vi "1. JKISM vs CSM.vi"() -> ()   [LabVIEW 2017]
doc: "### 1. JKISM vs CSM.vi\n\n#### Overview\n\nCSM 是仿照 JKISM 逻辑设计的 LabVIEW 程序开发框架，两个框架都使用基于字符串的消息队列来实现核心逻辑。本示例用于演示CSM基于JKISM的拓展。\n\n#### Introduction\n\n本示例比较 JKISM 框架和 CSM 框架之间的代码。两个框架都使用基于字符串的消息队列来实现核心状态机。\n\n#### Steps\n\n基于 JKISM，CSM 具有以下主要扩展功能，让我们逐步解释：\n\n- Step1: CSM是一个程序框架因此它需要模块的名称\n- Step2：重新设计了核心字符串解析引擎。\n- Step2.1 JKISM 使用 Parse State Queue.vi，它只输出下一个状态队列及其对应的参数（位于 >> 之后），主要用作“出队元素”。\n- Step2.2 CSM 使用 Parse State Queue++.vi 额外添加了以下主要功能：\n \\- 基于状态队列输入自动创建/处理/销毁队列/用户事件机制，因此用户只需给出相应的高级字符串消息。\n \\- 模块间/VI 间的消息可以被传输。\n \\- 额外的输入，如 Dequeue Timeout、Response Timeout 和 Allowed Messages，用于实现更高级的功能。\n- Step3：CSM 添加了一个内部状态调试日志 history.vi 用于更好的调试和记录，状态历史可以直接显示在前面板上。\n- Step4：CSM 定义了一系列字符串语法来实现本地/模块间消息传输，例如同步消息、异步消息、状态创建/注册/注销等。\n- Step4.1: JKISM 只定义了本地状态的轮转。它可以携带一个参数以及注释。\n- Step4.2: CSM是一个软件框架，因此它定义了模块。以及模块之间的消息通讯。\n- Step5: CSM 定义了一些基础的状态，用于处理模块之间通讯的逻辑行为。\n- Step5.1: \"Critical Error\" 用于处理一些无法恢复的错误。\n- Step5.2: \"Target Timeout Error\" 用于处理模块消息通讯超时的错误。\n- Step5.3: \"Target Error\" 用于处理模块不存在的错误。\n- STEP5.4: \"Async Response\" 用于处理异步消息的回复。\n- Step5.5：”Response\" 用于处理同步消息的回复。\n- Step5.6: \"Async Message Posted\" 用于处理异步消息发送后的操作。\n- Step5.7:(optional) \"Events: Register\" 和 \"Events: Unregister\" 中使用的消息事件，用于触发带有Event Structure的CSM模块跳出。\n- Step5.7:(optional) \"<New State Notifier Event>\" 配合Step5.7实现在外部消息到来后，跳出事件结构等待\n- Step5.8:(optional) CSM推荐使用 API 分组提供对外的接口，但是实际上所有的分支都可以使用消息调用。\n- Step6. CSM额外定义了\"Msg/Rsp's CSM\" 用于定位外部消息、状态的来源模块\n- Step7. 额外的消息信息，如Response的源消息名称、源参数等，可以由此获得。\n- Step8. CSM 预置了消息返回.\n- Step9：CSM 扩展了调试工具，详情请参阅选板 CSM->CSM Debug Tools。"
uses:
  user.lib/_NEVSTOP/Communicable State Machine(CSM)/AdvanceAPI/CSM - Revert Arguments-Safe String.vi
  user.lib/_NEVSTOP/Communicable State Machine(CSM)/AdvanceAPI/CSM - Make String Arguments Safe.vi
  user.lib/_NEVSTOP/Communicable State Machine(CSM)/AdvanceAPI/CSM - Break Down Multiple States String.vi
  user.lib/_NEVSTOP/Communicable State Machine(CSM)/AdvanceAPI/CSM - Compact Multiple States.vi
  user.lib/_NEVSTOP/Communicable State Machine(CSM)/AdvanceAPI/CSM - Keywords.vi
  user.lib/_NEVSTOP/Communicable State Machine(CSM)/_Shared/Trim Single-line Text.vi
  user.lib/_NEVSTOP/Communicable State Machine(CSM)/Communicable State Machine.lvlib
panel:
  out "State History":string
  in  "Exit":bool
  # "#CSM-Example Overview\n\nCSM 是仿照 JKISM 逻辑设计的 LabVIEW 程序开发框架，两个框架都使用基于字符串的消息队列来实现核心逻辑。本示例用于演示CSM基于JKISM的拓展。"
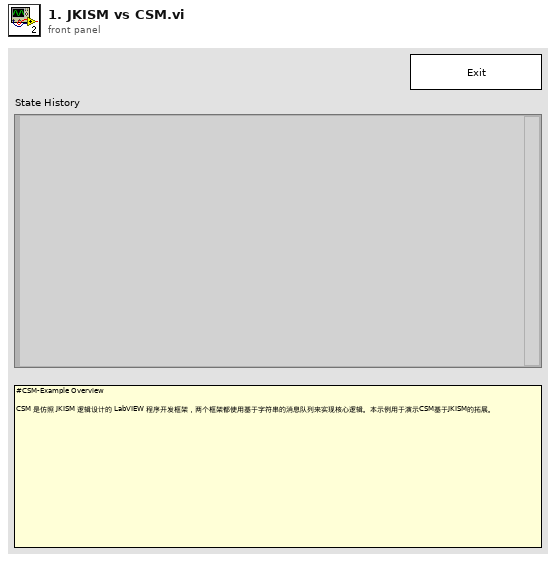
[diagram p1: front panel]
types:
  T1 = enum32{"Invalid", "Standard", "Closed", "Hidden", "Minimized", "Maximized"}
  T2 = enum32{"invalid app kind", "Development System", "Run Time System", "Student Edition", "Embedded LabVIEW", "Evaluation", "Custom"}
  T3 = cluster{"Core":cluster{"Current VI Reference":refnum<vi>, "Close Panel on Exit?":bool}, "Your Boolean data":bool, "Your string data":string}
  T4 = cluster{"Current VI Reference":refnum<vi>, "Close Panel on Exit?":bool}
  T5 = typedef "Communicable State Machine.lvlib/_CSM_Response Source Message.ctl" = cluster{"‘State":string, "’Arguments":string, "’Error":errorcluster}
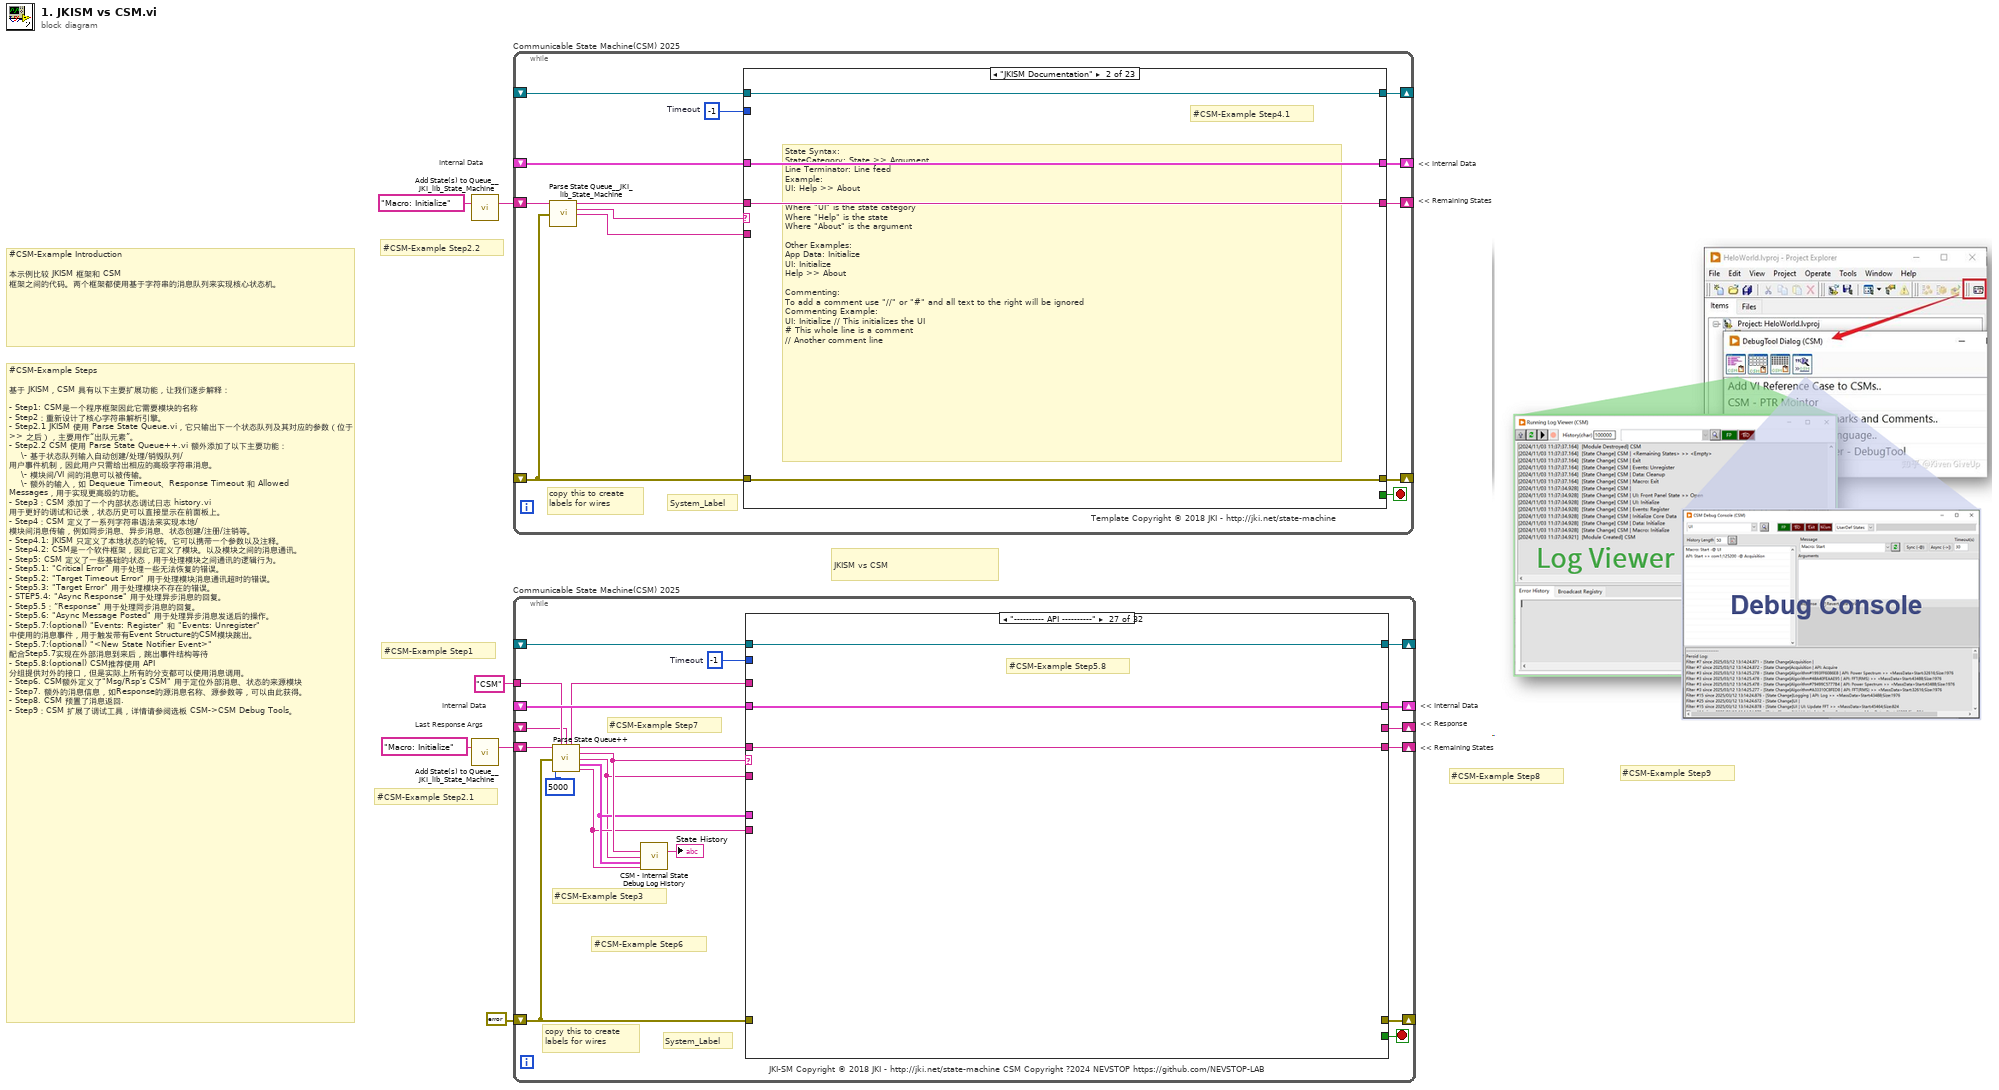
[diagram p0: block diagram]
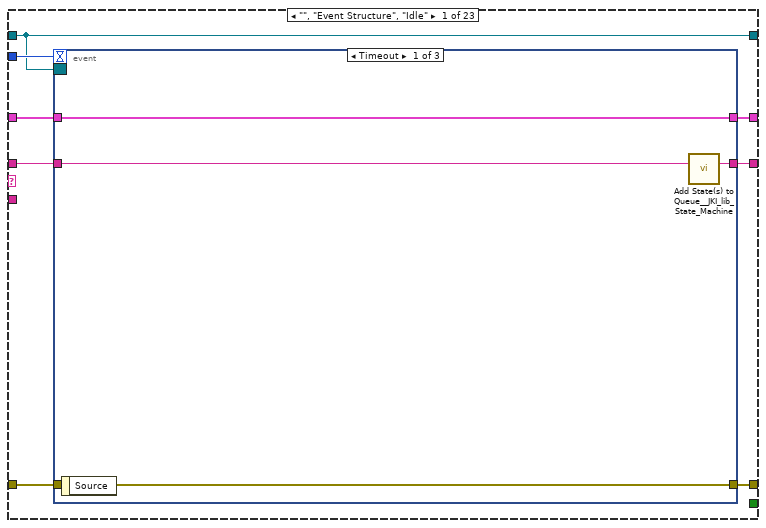
[diagram p2: hidden frame]
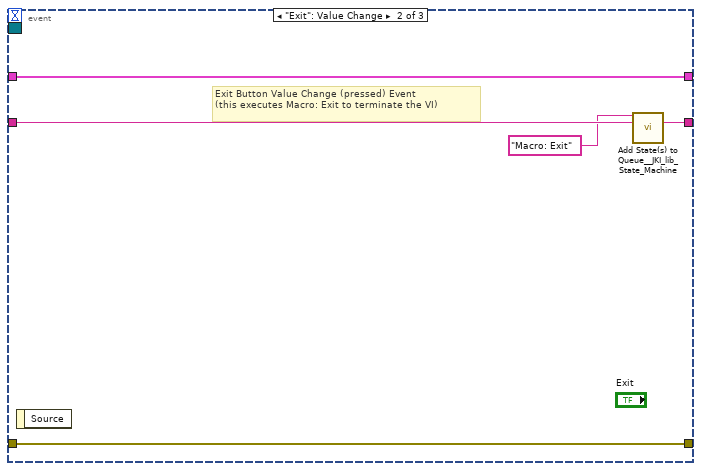
[diagram p3: hidden frame]
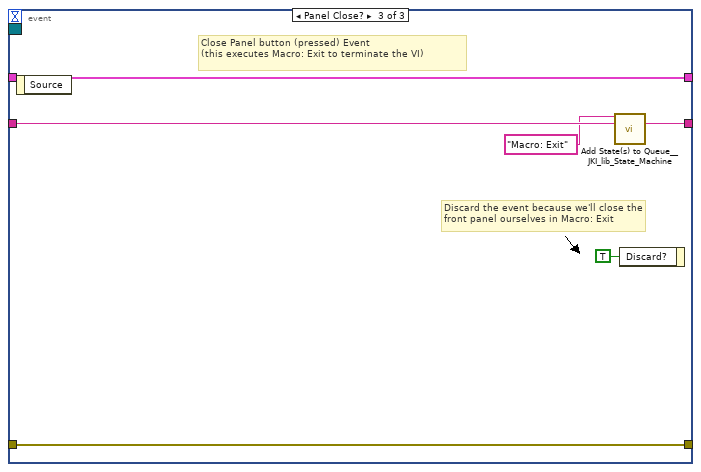
[diagram p4: hidden frame]
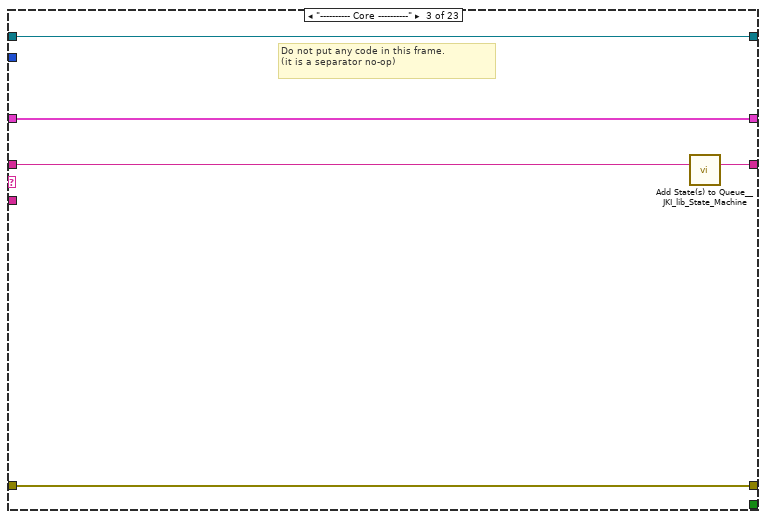
[diagram p5: hidden frame]
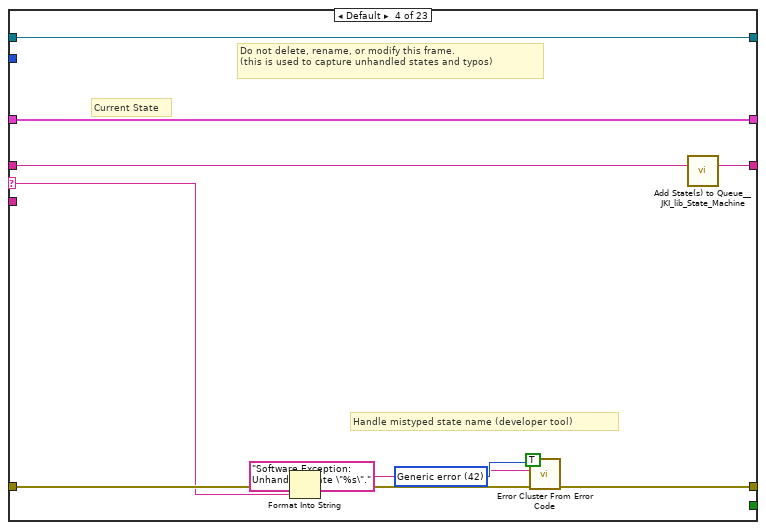
[diagram p6: hidden frame]
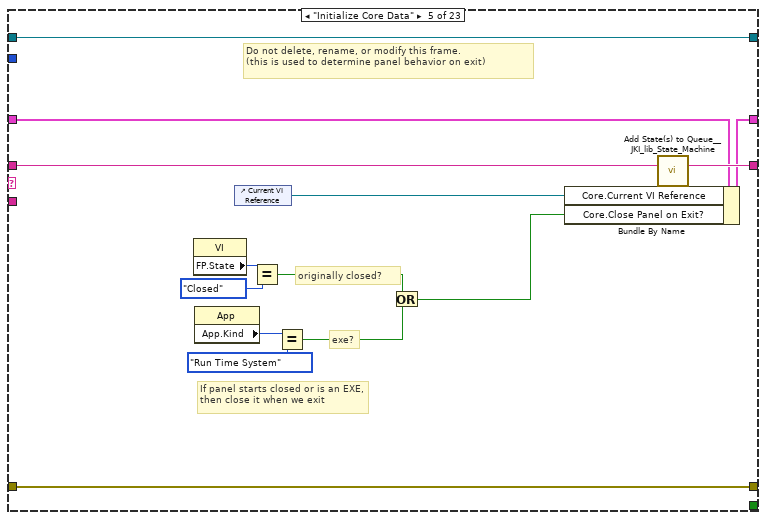
[diagram p7: hidden frame]
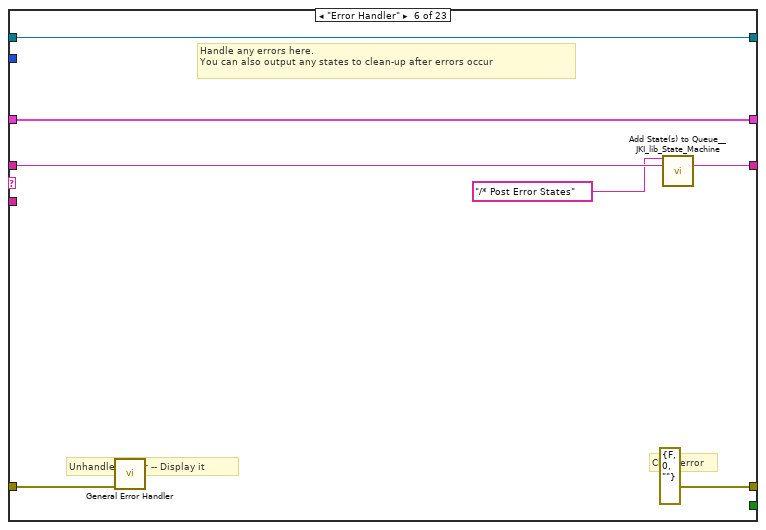
[diagram p8: hidden frame]
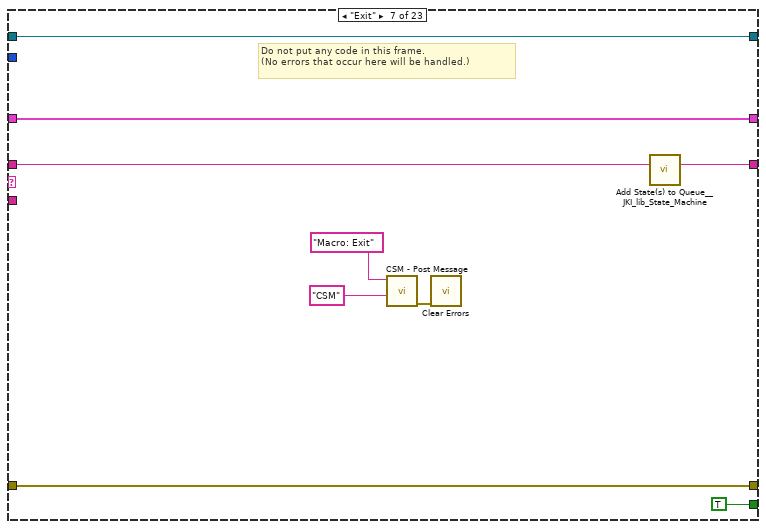
[diagram p9: hidden frame]
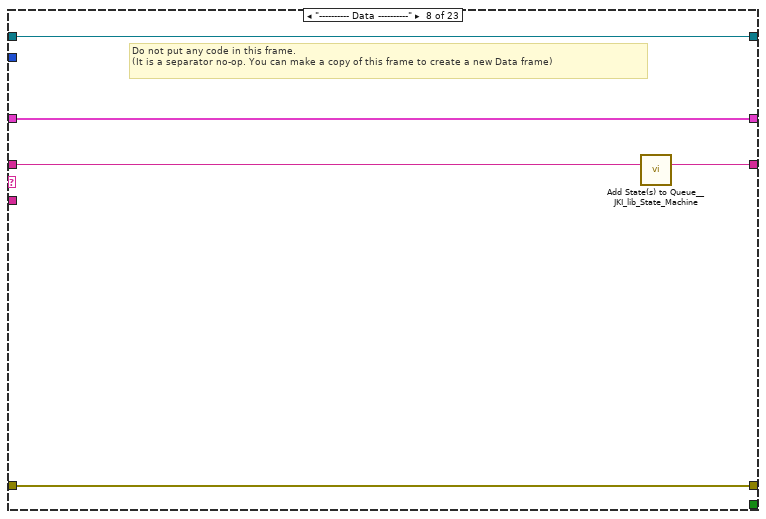
[diagram p10: hidden frame]
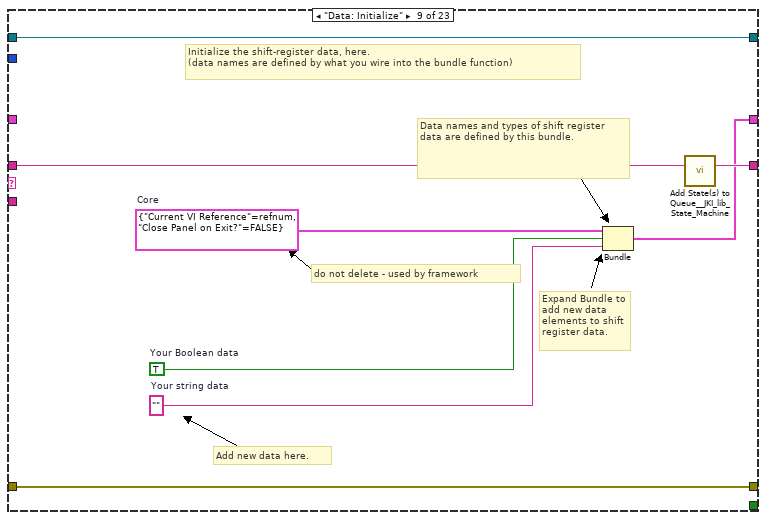
[diagram p11: hidden frame]
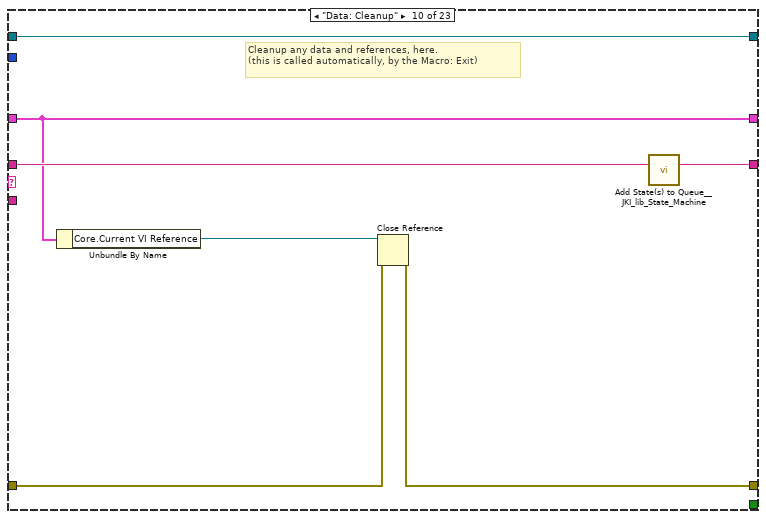
[diagram p12: hidden frame]
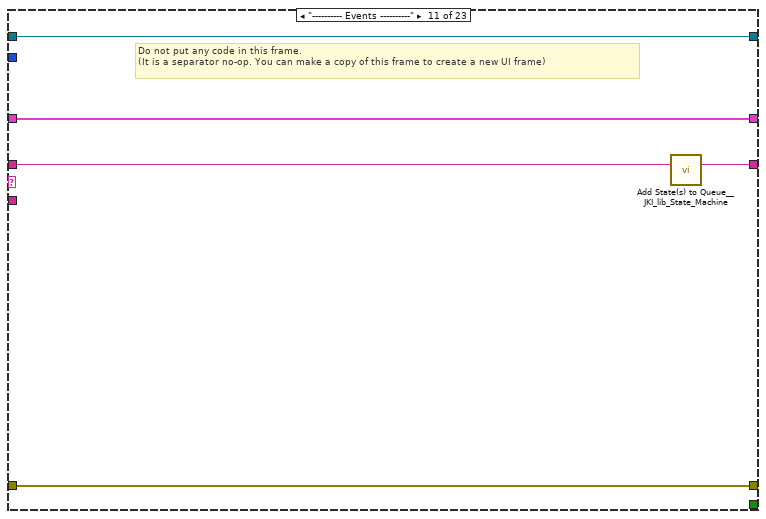
[diagram p13: hidden frame]
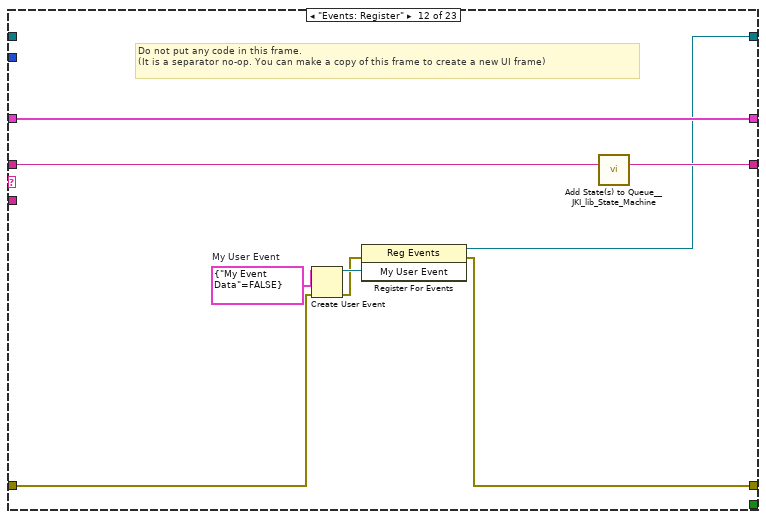
[diagram p14: hidden frame]
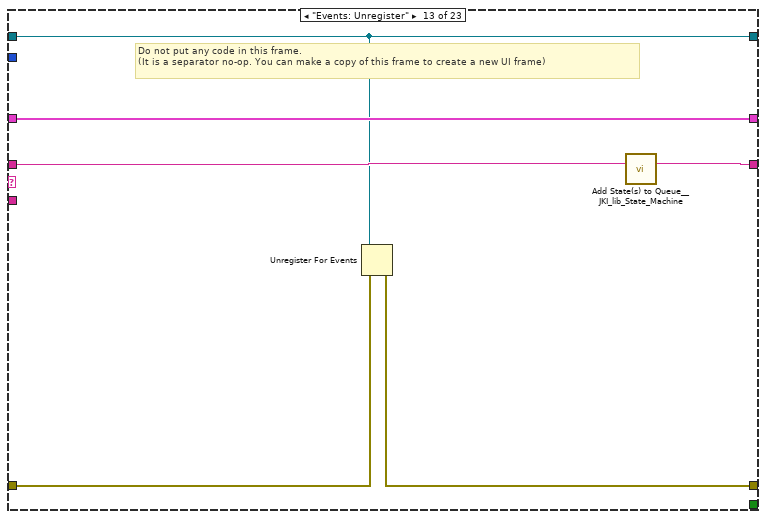
[diagram p15: hidden frame]
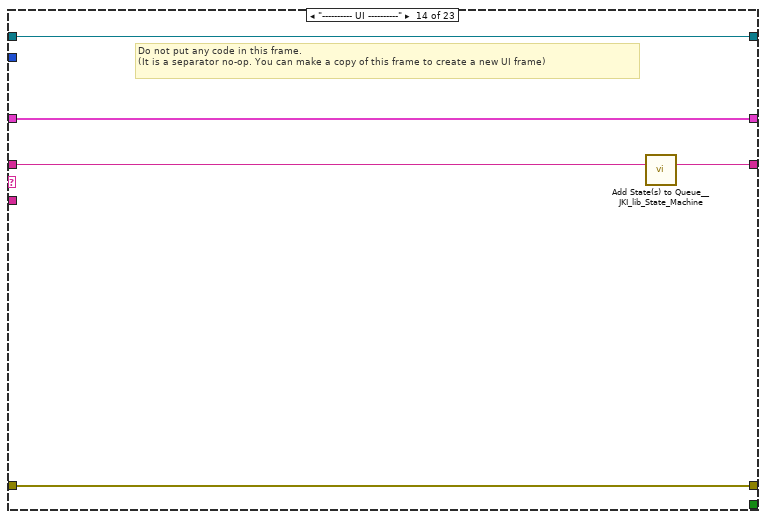
[diagram p16: hidden frame]
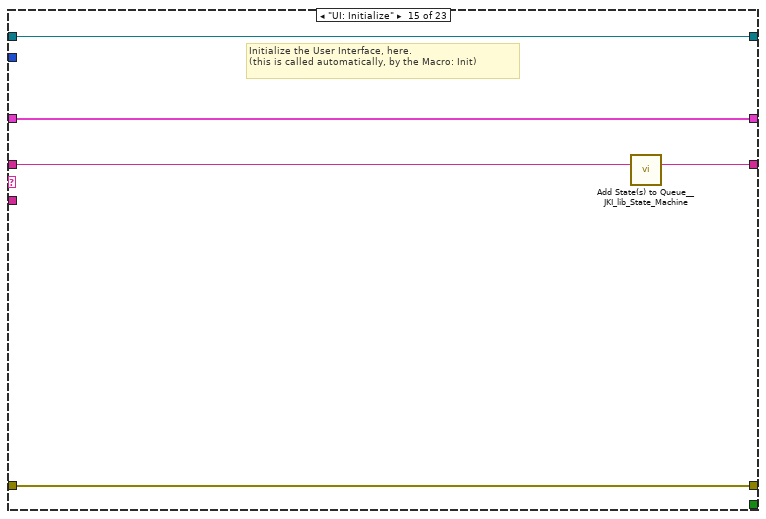
[diagram p17: hidden frame]
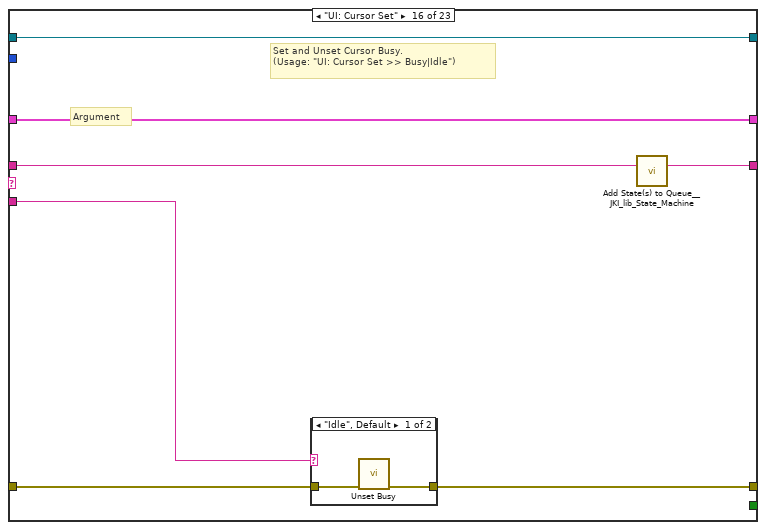
[diagram p18: hidden frame]
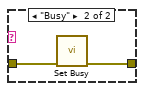
[diagram p19: hidden frame]
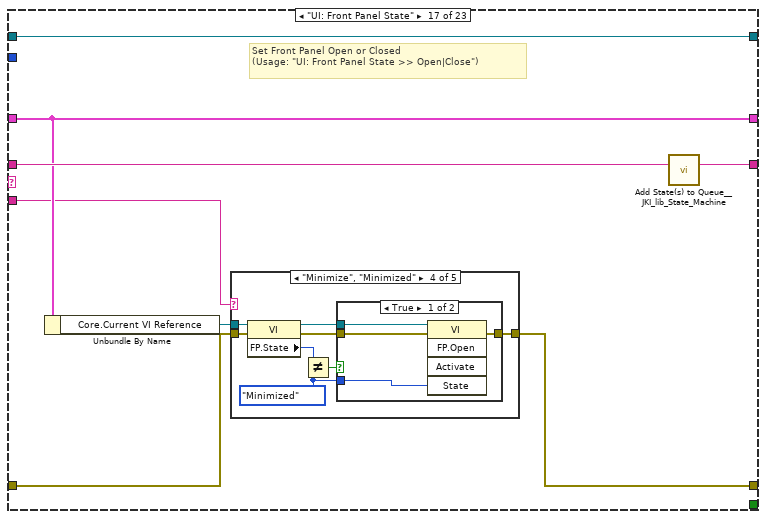
[diagram p20: hidden frame]
diagram:
  # "#CSM-Example Step9"
  # "#CSM-Example Step8"
  # "#CSM-Example Step2.2"
  # "#CSM-Example Step2.1"
  # "#CSM-Example Step1"
  # "#CSM-Example Steps\n\n基于 JKISM，CSM 具有以下主要扩展功能，让我们逐步解释：\n\n- Step1: CSM是一个程序框架因此它需要模块的名称\n- Step2：重新设计了核心字符串解析引擎。\n- Step2.1 JKISM 使用 Parse State Queue.vi，它只输出下一个状态队列及其对应的参数（位于 >> 之后），主要用作“出队元素”。\n- Step2.2 CSM 使用 Parse State Queue++.vi 额外添加了以下主要功能：\n    \\- 基于状态队列输入自动创建/处理/销毁队列/用户事件机制，因此用户只需给出相应的高级字符串消息。\n    \\- 模块间/VI 间的消息可以被传输。\n    \\- 额外的输入，如 Dequeue Timeout、Response Timeout 和 Allowed Messages，用于实现更高级的功能。\n- Step3：CSM 添加了一个内部状态调试日志 history.vi 用于更好的调试和记录，状态历史可以直接显示在前面板上。\n- Step4：CSM 定义了一系列字符串语法来实现本地/模块间消息传输，例如同步消息、异步消息、状态创建/注册/注销等。\n- Step4.1: JKISM 只定义了本地状态的轮转。它可以携带一个参数以及注释。\n- Step4.2: CSM是一个软件框架，因此它定义了模块。以及模块之间的消息通讯。\n- Step5: CSM 定义了一些基础的状态，用于处理模块之间通讯的逻辑行为。\n- Step5.1: \"Critical Error\" 用于处理一些无法恢复的错误。\n- Step5.2: \"Target Timeout Error\" 用于处理模块消息通讯超时的错误。\n- Step5.3: \"Target Error\" 用于处理模块不存在的错误。\n- STEP5.4: \"Async Response\" 用于处理异步消息的回复。\n- Step5.5：”Response\" 用于处理同步消息的回复。\n- Step5.6: \"Async Message Posted\" 用于处理异步消息发送后的操作。\n- Step5.7:(optional) \"Events: Register\" 和 \"Events: Unregister\" 中使用的消息事件，用于触发带有Event Structure的CSM模块跳出。\n- Step5.7:(optional) \"<New State Notifier Event>\" 配合Step5.7实现在外部消息到来后，跳出事件结构等待\n- Step5.8:(optional) CSM推荐使用 API 分组提供对外的接口，但是实际上所有的分支都可以使用消息调用。\n- Step6. CSM额外定义了\"Msg/Rsp's CSM\" 用于定位外部消息、状态的来源模块\n- Step7. 额外的消息信息，如Response的源消息名称、源参数等，可以由此获得。\n- Step8. CSM 预置了消息返回.\n- Step9：CSM 扩展了调试工具，详情请参阅选板 CSM->CSM Debug Tools。"
  # "#CSM-Example Introduction\n\n本示例比较 JKISM 框架和 CSM 框架之间的代码。两个框架都使用基于字符串的消息队列来实现核心状态机。"
  # "JKISM vs CSM"
  # "<< Internal Data"
  # "<< Remaining States"
  # "Internal Data"
  # "Last Response Args"
  # "Internal Data"
  # "<< Internal Data"
  # "<< Response"
  # "<< Remaining States"
  n1 = call <vilib>:"Add State(s) to Queue__JKI_lib_State_Machine.vi"("State(s) in (\"\")"="Macro: Initialize") -> ("States Out"=w6:string)  [unwired: 14 in]
  n2 = call <vilib>:"Add State(s) to Queue__JKI_lib_State_Machine.vi"("State(s) in (\"\")"="Macro: Initialize" ("Init State(\"Macro: Initialize\")")) -> ("States Out"=w1:string)  [unwired: 14 in]
  n3 = while "Communicable State Machine(CSM) 2025" {
    shift-right: [w12] -> _
    shift-left: _ -> [w11]
    shift-right: [w15] -> _
    shift-left: _ -> [w9]
    shift-right: [w14] -> _
    shift-left: w6 -> [w16]
    shift-right: [w8] -> _
    shift-left: _ -> [w7]
    stop <- w13 stop-if-true
    w10 = -1  # Timeout
    # "copy this to create labels for wires"
    # "System_Label"
    # "Template Copyright © 2018 JKI - http://jki.net/state-machine"
    n4 = call <vilib>:"Parse State Queue__JKI_lib_State_Machine.vi"("State Queue"=w16, "Error In (no error)"=w9) -> ("Remaining States"=w18:string, "Current State"=w19:string, "Arguments"=w17:string)  [unwired: 11 in]
    n5 = case shown="\"JKISM Documentation\"" w19 {
      selector: w19 -> [_ _ _ w53 _ _ _ _ _ _ _ _ _ _ _ _ _ _ _ _ _ _ _]
      tunnel: w18 -> [w27 w44 w51 w57 w77 w84 w93 w98 w106 w113 w118 w127 w133 w138 w143 w150 w162 w232 w238 w249 w254 w259 w264]
      tunnel: w17 -> [_ _ _ _ _ _ _ _ _ _ _ _ _ _ _ w145 w156 _ _ _ _ _ _]
      tunnel: w11 -> [w25 w45 w48 w55 w70 w81 w91 w95 _ w108 w115 w125 w131 w135 w141 w148 w158 w229 w235 w246 w251 w256 w261]
      tunnel: [w24 w43 w49 w59 w74 errorcluster {"status"=FALSE, "code"=0, "source"=""} ("error out") w90 w96 w103 w109 w116 w119 w128 w136 w140 w146 w159 w230 w236 w247 w252 w257 w262] -> w15
      tunnel: w9 -> [w23 w43 w49 w58 w74 w80 w90 w96 w103 w110 w116 w121 w129 w136 w140 w147 w160 w230 w236 w247 w252 w257 w262]
      tunnel: [w26 w44 w50 w56 w76 w83 w92 w97 w105 w112 w117 w126 w132 w137 w142 w149 w161 w231 w237 w248 w253 w258 w263] -> w14
      tunnel: [_ _ _ _ _ _ TRUE _ _ _ _ _ _ _ _ _ _ _ _ _ _ _ _] -> w13
      tunnel: [w22 w45 w48 w55 w75 w81 w91 w95 w104 w108 w115 w125 w131 w135 w141 w148 w158 w229 w235 w246 w251 w256 w261] -> w12
      tunnel: w10 -> [w21 _ _ _ _ _ _ _ _ _ _ _ _ _ _ _ _ _ _ _ _ _ _]
      tunnel: [w20 w46 w47 w52 w64 w78 w88 w94 w99 w107 w114 w122 w130 w134 w139 w144 w155 w228 w233 w239 w250 w255 w260] -> w8
      tunnel: w7 -> [w20 w46 w47 w52 w64 w78 w88 w94 w99 w107 w114 _ w130 w134 w139 w144 w155 w228 w233 w239 w250 w255 w260]
      frame "", "Event Structure", "Idle" {
        n6 = event shown="[0] Timeout" {
          selector: w20 -> [_ _ _]
          dyn-events: _ -> [_ _ _]
          timeout: w21 -> [_ _ _]
          tunnel: w27 -> [w31 w36 w42]
          tunnel: [w30 w35 w41] -> w26
          tunnel: w25 -> [w28 w33 w39]
          tunnel: [w29 w34 w40] -> w24
          tunnel: w23 -> [w29 w34 w40]
          tunnel: [w28 w33 w39] -> w22
          event Timeout {
            n7 = event-data() -> ()  [unwired: 1 in, 1 out]
            n8 = call <vilib>:"Add State(s) to Queue__JKI_lib_State_Machine.vi"("State(s) in (\"\")"=w31) -> ("States Out"=w30:string)  [unwired: 14 in]
          }
          event "Exit": Value Change {
            # "Exit Button Value Change (pressed) Event\n(this executes Macro: Exit to terminate the VI)"
            n9 = event-data() -> ()  [unwired: 1 in, 1 out]
            n10 = call <vilib>:"Add State(s) to Queue__JKI_lib_State_Machine.vi"("State(s) in Front (\"\")"="Macro: Exit", "State(s) in (\"\")"=w36) -> ("States Out"=w35:string)  [unwired: 13 in]
          }
          event Panel Close? {
            # "Discard the event because we'll close the front panel ourselves in Macro: Exit"
            # "Close Panel button (pressed) Event\n(this executes Macro: Exit to terminate the VI)"
            n11 = event-data() -> ()  [unwired: 1 in, 1 out]
            n12 = call <vilib>:"Add State(s) to Queue__JKI_lib_State_Machine.vi"("State(s) in Front (\"\")"="Macro: Exit", "State(s) in (\"\")"=w42) -> ("States Out"=w41:string)  [unwired: 13 in]
            n13 = event-data("Discard?"=TRUE) -> ()  [unwired: 1 in, 1 out]
          }
        }
      }
      frame "JKISM Documentation" {
        # "State Syntax:\nStateCategory: State >> Argument\nLine Terminator: Line feed\nExample:\nUI: Help >> About\n\nWhere \"UI\" is the state category\nWhere \"Help\" is the state\nWhere \"About\" is the argument\n\nOther Examples:\nApp Data: Initialize\nUI: Initialize\nHelp >> About\n\nCommenting:\nTo add a comment use \"//\" or \"#\" and all text to the right will be ignored\nCommenting Example:\nUI: Initialize // This initializes the UI\n# This whole line is a comment\n// Another comment line"
        # "#CSM-Example Step4.1"
      }
      frame "---------- Core ----------" {
        # "Do not put any code in this frame.\n(it is a separator no-op)"
        n14 = call <vilib>:"Add State(s) to Queue__JKI_lib_State_Machine.vi"("State(s) in (\"\")"=w51) -> ("States Out"=w50:string)  [unwired: 14 in]
      }
      frame Default {
        w62 = 42 items=["No error", "Argument error", "Memory is full", "Out of zone", "End of file", "File already open", "Generic file I/O error", "File not found", "File permission error", "Disk is full", "Duplicate path", "Too many files open", "System feature not enabled", "Resource file not found", "Cannot add resource", "Resource not found", "Image not found", "Image memory error", "Pen does not exist", "Config type invalid", "Config token not found", "Config parse error", "Config memory error", "Bad external code format", "Bad external code offset", "External code not present", "Null window", "Destroy window error", "Null menu", "Print aborted", "Bad print record", "Print driver error", "Windows error during printing", "Memory error during printing", "Print dialog error", "Generic print error", "Invalid device refnum", "Device not found", "Device parameter error", "Device unit error", "Cannot open device", "Device call aborted", "Generic error", "Cancelled by user", "Object ID too low", "Object ID too high", "Object not in heap", "Unknown heap", "Unknown object (invalid DefProc)", "Unknown object (DefProc not in table)", "Message out of range", "Invalid (null) method", "Unknown message", "Manager call not supported", "Bad address", "Network operation in progress", "Network operation timed out", "Connection is busy", "Network attribute not supported", "Network error", "Address in use", "System out of memory", "Connection aborted", "Connection refused", "Not connected", "Already connected", "Connection closed", "Initialization error (interapplication manager)", "Bad occurrence", "Wait on unbound occurrence handler", "Occurrence queue overflow", "Datalog type conflict", "Unused", "Unrecognized type (interapplication manager)", "Memory corrupt", "Failed to make temporary DLL", "Old CIN version", "Drag socket not found", "Failed to load drop-object", "Failed to register OLE object", "Failed to release OLE object", "Format specifier type mismatch", "Unknown format specifier", "Too few format specifiers", "Too many format specifiers", "Scan failed", "Newer CIN version", "Error converting to variant", "Runtime menu error", "Password tampered", "Variant attribute not found", "Incompatible variant data type", "Event data is not available", "Event Store is not present", "Occurrence is not found", "Event Queue is not created", "Event info is not available", "Refnum passed is NULL", "Error retrieving Class GUID", "Error retrieving CoClass GUID", "Error retrieving TypeLib GUID.", "Bad built application magic bytes.", "Specific driver is different from the specific driver associated with the Logical Name.", "There is no session opened to the class driver.", "Max Error", "MAX - Error with config objects", "MAX - Error loading configuration", "MAX - Group not supported"]
        # "Current State"
        # "Do not delete, rename, or modify this frame.\n(this is used to capture unhandled states and typos)"
        # "Handle mistyped state name (developer tool)"
        n15 = Format Into String(format string="Software Exception: Unhandled State \"%s\"." ("message"), error in=w58, w53) -> (resulting string=w61:string, error out=w60:errorcluster)  [unwired: 1 in]
        n16 = call <vilib>:"Error Cluster From Error Code.vi"("show call chain? (False)"=TRUE, "error in (no error)"=w60, "error message (\"\")"=w61, "error code (0)"=w62) -> ("error out"=w59:errorcluster)  [unwired: 5 in]
        n17 = call <vilib>:"Add State(s) to Queue__JKI_lib_State_Machine.vi"("State(s) in (\"\")"=w57) -> ("States Out"=w56:string)  [unwired: 14 in]
      }
      frame "Initialize Core Data" {
        # "Do not delete, rename, or modify this frame.\n(this is used to determine panel behavior on exit)"
        # "originally closed?"
        # "exe?"
        # "If panel starts closed or is an EXE, then close it when we exit"
        n18 = property class="VI"() -> ("FP.State"=w67:T1)  [unwired: 2 in, 2 out]
        n19 = property class="App"() -> ("App.Kind"=w73:T2)  [unwired: 2 in, 2 out]
        n20 = control-ref of="Current VI Reference"() -> (w68:refnum<vi>)
        n21 = Equal?(x=w67, y=T1."Closed" ("Front Panel Window:State")) -> (x = y?=w65:bool)
        n22 = Equal?(x=w73, y=T2."Run Time System" ("Application:Kind")) -> (x = y?=w71:bool)
        n23 = Or(x=w65, y=w71) -> (x .or. y?=w69:bool)
        n24 = Bundle By Name(cluster=w70, "Core.Current VI Reference"=w68, "Core.Close Panel on Exit?"=w69) -> (w75:T3)
        n25 = call <vilib>:"Add State(s) to Queue__JKI_lib_State_Machine.vi"("State(s) in (\"\")"=w77) -> ("States Out"=w76:string)  [unwired: 14 in]
      }
      frame "Error Handler" {
        # "Unhandled Error -- Display it"
        # "Handle any errors here.\nYou can also output any states to clean-up after errors occur"
        # "Clear error"
        n26 = call <vilib>:"General Error Handler.vi"("error in (no error)"=w80) -> ()  [unwired: 10 in, 5 out]
        n27 = call <vilib>:"Add State(s) to Queue__JKI_lib_State_Machine.vi"("State(s) in Front (\"\")"="/* Post Error States", "State(s) in (\"\")"=w84) -> ("States Out"=w83:string)  [unwired: 13 in]
      }
      frame "Exit" {
        # "Do not put any code in this frame.\n(No errors that occur here will be handled.)"
        n28 = call "CSM - Post Message.vi"("Target Module"="CSM", "State"="Macro: Exit") -> ("error out"=w86:errorcluster)  [unwired: 9 in]
        n29 = call <vilib>:"Clear Errors.vi"("error in (no error)"=w86) -> ()  [unwired: 5 in, 2 out]
        n30 = call <vilib>:"Add State(s) to Queue__JKI_lib_State_Machine.vi"("State(s) in (\"\")"=w93) -> ("States Out"=w92:string)  [unwired: 14 in]
      }
      frame "---------- Data ----------" {
        # "Do not put any code in this frame.\n(It is a separator no-op. You can make a copy of this frame to create a new Data frame)"
        n31 = call <vilib>:"Add State(s) to Queue__JKI_lib_State_Machine.vi"("State(s) in (\"\")"=w98) -> ("States Out"=w97:string)  [unwired: 14 in]
      }
      frame "Data: Initialize" {
        w100 = T4 {"Current VI Reference"=refnum, "Close Panel on Exit?"=FALSE}  # Core
        w102 = TRUE  # Your Boolean data
        w101 = ""  # Your string data
        # "do not delete - used by framework"
        # "Expand Bundle to add new data elements to shift register data."
        # "Add new data here."
        # "Data names and types of shift register data are defined by this bundle."
        # "Initialize the shift-register data, here.\n(data names are defined by what you wire into the bundle function)"
        n32 = Bundle("Core"=w100, "Your Boolean data"=w102, "Your string data"=w101) -> (w104:T3)  [unwired: 1 in]
        n33 = call <vilib>:"Add State(s) to Queue__JKI_lib_State_Machine.vi"("State(s) in (\"\")"=w106) -> ("States Out"=w105:string)  [unwired: 14 in]
      }
      frame "Data: Cleanup" {
        # "Cleanup any data and references, here.\n(this is called automatically, by the Macro: Exit)"
        n34 = Unbundle By Name(w108) -> ("Core.Current VI Reference"=w111:refnum<vi>)
        n35 = Close Reference(reference=w111, error in (no error)=w110) -> (error out=w109:errorcluster)
        n36 = call <vilib>:"Add State(s) to Queue__JKI_lib_State_Machine.vi"("State(s) in (\"\")"=w113) -> ("States Out"=w112:string)  [unwired: 14 in]
      }
      frame "---------- Events ----------" {
        # "Do not put any code in this frame.\n(It is a separator no-op. You can make a copy of this frame to create a new UI frame)"
        n37 = call <vilib>:"Add State(s) to Queue__JKI_lib_State_Machine.vi"("State(s) in (\"\")"=w118) -> ("States Out"=w117:string)  [unwired: 14 in]
      }
      frame "Events: Register" {
        w123 = cluster{"My Event Data":bool} {"My Event Data"=FALSE}  # My User Event
        # "Do not put any code in this frame.\n(It is a separator no-op. You can make a copy of this frame to create a new UI frame)"
        n38 = Create User Event(user event datatype=w123, error in=w121) -> (user event=w124:refnum<user-event>, error out=w120:errorcluster)
        n39 = register-events(error in=w120, w124) -> (reference out=w122:refnum<event-registration>, error out=w119:errorcluster)  [unwired: 1 in]
        n40 = call <vilib>:"Add State(s) to Queue__JKI_lib_State_Machine.vi"("State(s) in (\"\")"=w127) -> ("States Out"=w126:string)  [unwired: 14 in]
      }
      frame "Events: Unregister" {
        # "Do not put any code in this frame.\n(It is a separator no-op. You can make a copy of this frame to create a new UI frame)"
        n41 = Unregister For Events(event registration refnum=w130, error in=w129) -> (error out=w128:errorcluster)
        n42 = call <vilib>:"Add State(s) to Queue__JKI_lib_State_Machine.vi"("State(s) in (\"\")"=w133) -> ("States Out"=w132:string)  [unwired: 14 in]
      }
      frame "---------- UI ----------" {
        # "Do not put any code in this frame.\n(It is a separator no-op. You can make a copy of this frame to create a new UI frame)"
        n43 = call <vilib>:"Add State(s) to Queue__JKI_lib_State_Machine.vi"("State(s) in (\"\")"=w138) -> ("States Out"=w137:string)  [unwired: 14 in]
      }
      frame "UI: Initialize" {
        # "Initialize the User Interface, here.\n(this is called automatically, by the Macro: Init)"
        n44 = call <vilib>:"Add State(s) to Queue__JKI_lib_State_Machine.vi"("State(s) in (\"\")"=w143) -> ("States Out"=w142:string)  [unwired: 14 in]
      }
      frame "UI: Cursor Set" {
        # "Argument"
        # "Set and Unset Cursor Busy.\n(Usage: \"UI: Cursor Set >> Busy|Idle\")"
        n45 = case shown="\"Idle\", Default" w145 {
          tunnel: w147 -> [w152 w154]
          tunnel: [w151 w153] -> w146
          frame "Idle", Default {
            n46 = call <vilib>:"Unset Busy.vi"("error in (no error)"=w152) -> ("error out"=w151:errorcluster)  [unwired: 10 in]
          }
          frame "Busy" {
            n47 = call <vilib>:"Set Busy.vi"("error in (no error)"=w154) -> ("error out"=w153:errorcluster)  [unwired: 9 in, 1 out]
          }
        }
        n48 = call <vilib>:"Add State(s) to Queue__JKI_lib_State_Machine.vi"("State(s) in (\"\")"=w150) -> ("States Out"=w149:string)  [unwired: 14 in]
      }
      frame "UI: Front Panel State" {
        # "Set Front Panel Open or Closed\n(Usage: \"UI: Front Panel State >> Open|Close\")"
        n49 = Unbundle By Name(w158) -> ("Core.Current VI Reference"=w157:refnum<vi>)
        n50 = case shown="\"Minimize\", \"Minimized\"" w156 {
          tunnel: w160 -> [w168 w183 w194 w207 w220]
          tunnel: [w170 w184 w196 w209 w222] -> w159
          tunnel: w157 -> [w169 w181 w195 w208 w221]
          frame "Open", "Standard", Default {
            w163 = T1."Standard" ("State")
            n51 = property class="VI"(reference=w169, error in=w168) -> (reference out=w166:refnum<vi>, error out=w167:errorcluster, "FP.State"=w165:T1)
            n52 = Not Equal?(x=w165, y=w163) -> (x != y?=w164:bool)
            n53 = case shown="True" w164 {
              tunnel: [w174 w176] -> w170
              tunnel: w167 -> [w173 w176]
              tunnel: w166 -> [w172 _]
              tunnel: w163 -> [w171 _]
              frame True {
                n54 = invoke class="VI" method="FP.Open"(reference=w172, error in=w173, "Activate"=TRUE, "State"=w171) -> (error out=w174:errorcluster)  [unwired: 1 in, 4 out]
              }
              frame False {
              }
            }
          }
          frame "Close", "Closed" {
            n55 = property class="VI"(reference=w181, error in=w183) -> (reference out=w180:refnum<vi>, error out=w182:errorcluster, "FP.State"=w178:T1)
            n56 = Not Equal?(x=w178, y=T1."Closed" ("Front Panel Window:State")) -> (x != y?=w177:bool)
            n57 = case shown="True" w177 {
              tunnel: [w185 w188] -> w184
              tunnel: w182 -> [w185 w187]
              tunnel: w180 -> [_ w186]
              frame False {
              }
              frame True {
                n58 = invoke class="VI" method="FP.Close"(reference=w186, error in=w187) -> (error out=w188:errorcluster)  [unwired: 1 in, 2 out]
              }
            }
          }
          frame "Hidden", "Hide" {
            w189 = T1."Hidden" ("State")
            n59 = property class="VI"(reference=w195, error in=w194) -> (reference out=w192:refnum<vi>, error out=w193:errorcluster, "FP.State"=w191:T1)
            n60 = Not Equal?(x=w191, y=w189) -> (x != y?=w190:bool)
            n61 = case shown="True" w190 {
              tunnel: [w200 w201] -> w196
              tunnel: w193 -> [w199 w201]
              tunnel: w192 -> [w198 _]
              tunnel: w189 -> [w197 _]
              frame True {
                n62 = invoke class="VI" method="FP.Open"(reference=w198, error in=w199, "State"=w197) -> (error out=w200:errorcluster)  [unwired: 2 in, 4 out]
              }
              frame False {
              }
            }
          }
          frame "Minimize", "Minimized" {
            w202 = T1."Minimized" ("State")
            n63 = property class="VI"(reference=w208, error in=w207) -> (reference out=w205:refnum<vi>, error out=w206:errorcluster, "FP.State"=w204:T1)
            n64 = Not Equal?(x=w204, y=w202) -> (x != y?=w203:bool)
            n65 = case shown="True" w203 {
              tunnel: [w213 w214] -> w209
              tunnel: w206 -> [w212 w214]
              tunnel: w205 -> [w211 _]
              tunnel: w202 -> [w210 _]
              frame True {
                n66 = invoke class="VI" method="FP.Open"(reference=w211, error in=w212, "State"=w210) -> (error out=w213:errorcluster)  [unwired: 2 in, 4 out]
              }
              frame False {
              }
            }
          }
          frame "Maximize", "Maximized" {
            w215 = T1."Maximized" ("State")
            n67 = property class="VI"(reference=w221, error in=w220) -> (reference out=w218:refnum<vi>, error out=w219:errorcluster, "FP.State"=w217:T1)
            n68 = Not Equal?(x=w217, y=w215) -> (x != y?=w216:bool)
            n69 = case shown="True" w216 {
              tunnel: [w226 w227] -> w222
              tunnel: w219 -> [w225 w227]
              tunnel: w218 -> [w224 _]
              tunnel: w215 -> [w223 _]
              frame True {
                n70 = invoke class="VI" method="FP.Open"(reference=w224, error in=w225, "State"=w223) -> (error out=w226:errorcluster)  [unwired: 2 in, 4 out]
              }
              frame False {
              }
            }
          }
        }
        n71 = call <vilib>:"Add State(s) to Queue__JKI_lib_State_Machine.vi"("State(s) in (\"\")"=w162) -> ("States Out"=w161:string)  [unwired: 14 in]
      }
      frame "---------- Macro ----------" {
        # "Do not put any code in this frame.\n(It is a separator no-op. You can make a copy of this frame to create a new Macro frame)"
        n72 = call <vilib>:"Add State(s) to Queue__JKI_lib_State_Machine.vi"("State(s) in (\"\")"=w232) -> ("States Out"=w231:string)  [unwired: 14 in]
      }
      frame "Macro: Initialize" {
        # "Initialization Macro\n(This is called once, when the VI starts)"
        n73 = call <vilib>:"Add State(s) to Queue__JKI_lib_State_Machine.vi"("State(s) in Front (\"\")"="Data: Initialize\nInitialize Core Data\nEvents: Register\nUI: Initialize\nUI: Front Panel State >> Open", "State(s) in (\"\")"=w238) -> ("States Out"=w237:string)  [unwired: 13 in]
      }
      frame "Macro: Exit" {
        # "Exit Macro\n(This is called once, when the VI exits)"
        n74 = Unbundle By Name(w246) -> ("Core.Close Panel on Exit?"=w245:bool)
        n75 = Select(t="UI: Front Panel State >> Close", s=w245, f="") -> (s? t:f=w242:string)
        n76 = call <vilib>:"Add State(s) to Queue__JKI_lib_State_Machine.vi"("State(s) in (\"\")"=w242, "State(s) at Back (\"\")"="Data: Cleanup\nEvents: Unregister\nExit") -> ("States Out"=w240:string)  [unwired: 13 in]
        n77 = call <vilib>:"Add State(s) to Queue__JKI_lib_State_Machine.vi"("State(s) in Front (\"\")"=w240, "State(s) in (\"\")"=w249) -> ("States Out"=w248:string)  [unwired: 13 in]
      }
      frame "---------- New Category ----------" {
        # "Template Separator\n(You can make a copy of, or modify, this frame)"
        n78 = call <vilib>:"Add State(s) to Queue__JKI_lib_State_Machine.vi"("State(s) in (\"\")"=w254) -> ("States Out"=w253:string)  [unwired: 14 in]
      }
      frame "New Category: 1" {
        # "Your code here.\n(You can make a copy of, or modify, this frame)"
        n79 = call <vilib>:"Add State(s) to Queue__JKI_lib_State_Machine.vi"("State(s) in (\"\")"=w259) -> ("States Out"=w258:string)  [unwired: 14 in]
      }
      frame "New Category: 2" {
        # "Your code here.\n(You can make a copy of, or modify, this frame)"
        n80 = call <vilib>:"Add State(s) to Queue__JKI_lib_State_Machine.vi"("State(s) in (\"\")"=w264) -> ("States Out"=w263:string)  [unwired: 14 in]
      }
    }
  }
  n81 = while "Communicable State Machine(CSM) 2025" {
    shift-right: [w280] -> _
    shift-left: _ -> [w279]
    shift-right: [w283] -> _
    shift-left: errorcluster {"status"=FALSE, "code"=0, "source"=""} ("error out") -> [w277]
    shift-right: [w282] -> _
    shift-left: w1 -> [w284]
    tunnel: "CSM" ("Name (\"\" to Use UUID)") -> [w272]
    shift-right: [w275] -> _
    shift-left: _ -> [w267]
    shift-right: [w274] -> _
    shift-left: _ -> [w273]
    stop <- w281 stop-if-true
    w278 = -1  # Timeout
    # "#CSM-Example Step7"
    # "#CSM-Example Step6"
    # "#CSM-Example Step3"
    # "copy this to create labels for wires"
    # "System_Label"
    # "JKI-SM Copyright © 2018 JKI - http://jki.net/state-machine CSM Copyright ?2024 NEVSTOP https://github.com/NEVSTOP-LAB"
    n82 = call "Parse State Queue++.vi"("State Queue"=w284, "Name (\"\" to Use UUID)"=w272, "Response Arguments"=w267, "Previous Error"=w277, "Response Timeout (-2 Use Global Settings)"=5000 ("Response Timeout(1000ms)")) -> ("Name Used"=w268:string, "Remaining States"=w285:string, "Current State"=w271:string, "Arguments"=w266:string, "Additional Information"=w270:T5, "Source CSM"=w269:string)  [unwired: 5 in]
    n83 = call "CSM - Internal State Debug Log History.vi"("State"=w271, "Arguments (\"\")"=w266, ">> Response Source Message >>"=w270, "Source (\"\")"=w269) -> ("Debug Log"=→"State History":string)  [unwired: 11 in]
    n84 = case shown="\"---------- API ----------\"" w271 {
      selector: w271 -> [_ _ _ w316 _ _ _ _ _ _ _ _ _ _ _ _ _ _ _ _ _ _ _ _ _ _ _ _ _ _ _ _]
      tunnel: w285 -> [w287 w308 w313 w322 w328 w334 w360 w368 w375 w385 w394 w407 w412 w416 w423 w429 w433 w440 w444 w448 w452 w458 w469 w533 w538 w549 w552 w556 w559 w563 w567 w571]
      tunnel: w266 -> [_ _ _ _ _ w332 w356 w363 w371 w379 _ _ _ _ _ _ _ _ _ _ _ w454 w464 _ _ _ _ _ _ _ _ _]
      tunnel: w279 -> [w293 w307 w310 w320 w327 w340 w361 w366 w373 w383 w393 w401 w410 w414 _ w425 w431 w439 w443 w446 w450 w456 w466 w531 w536 w547 w551 w555 w558 w561 w565 w569]
      tunnel: [w292 _ w311 w314 w329 errorcluster {"status"=FALSE, "code"=0, "source"=""} ("error out") w353 w362 w369 w382 _ _ _ _ _ w426 _ w434 w442 _ _ w455 w467 _ _ _ _ _ _ _ _ _] -> w283
      tunnel: w277 -> [w286 _ w311 w315 w329 w338 w354 w364 w370 _ _ _ _ _ _ _ _ _ _ _ _ _ _ _ _ _ _ _ _ _ _ _]
      tunnel: [w294 w308 w312 w321 w328 w336 w359 w367 w374 w386 w394 w406 w411 w415 w422 w428 w432 w440 w444 w447 w451 w457 w468 w532 w537 w548 w552 w556 w559 w562 w566 w570] -> w282
      tunnel: [_ _ _ _ _ _ TRUE _ _ _ _ _ TRUE _ _ _ _ _ _ _ _ _ _ _ _ _ _ _ _ _ _ _] -> w281
      tunnel: [w291 w307 w310 w320 w327 w340 w361 w366 w373 w384 w393 w405 w410 w414 w421 w425 w431 w439 w443 w446 w450 w456 w466 w531 w536 w547 w551 w555 w558 w561 w565 w569] -> w280
      tunnel: w278 -> [w289 _ _ _ _ _ _ _ _ _ _ _ _ _ _ _ _ _ _ _ _ _ _ _ _ _ _ _ _ _ _ _]
      tunnel: w269 -> [_ _ _ _ _ w331 _ _ _ w380 _ _ _ _ _ _ _ _ _ _ _ _ _ _ _ _ _ _ _ _ _ _]
      tunnel: w270 -> [_ _ _ _ _ w330 _ _ _ w381 _ _ _ _ _ _ _ _ _ _ _ _ _ _ _ _ _ _ _ _ _ _]
      tunnel: [_ _ _ "" w323 _ _ _ _ _ _ _ _ _ _ _ _ _ _ _ _ _ _ _ _ _ _ "API1 Response" _ _ _ _] -> w275
      tunnel: [w290 w306 w309 w318 w326 w339 w357 w365 w372 w387 w392 w395 w408 w413 w417 w424 w430 w438 w441 w445 w449 w453 w463 w530 w534 w540 w550 w554 w557 w560 w564 w568] -> w274
      tunnel: w273 -> [w290 w306 w309 w318 w326 w339 w357 w365 w372 w387 w392 w395 w408 w413 w417 w424 w430 _ w441 w445 w449 w453 w463 w530 w534 w540 w550 w554 w557 w560 w564 w568]
      tunnel: w268 -> [_ _ _ w317 _ _ w355 _ _ _ _ _ _ _ _ _ _ w437 _ _ _ _ _ _ _ _ _ _ _ _ _ _]
      frame "", "Event Structure", "Idle" {
        n85 = call "Timeout Selector.vi"("Remaining States"=w287, "Timeout Expected"=w289) -> ("Timeout"=w288:i32)  [unwired: 5 in]
        n86 = event shown="[1] <New State Notifier Event>: User Event" {
          selector: w290 -> [_ _ _]
          dyn-events: _ -> [_ _ _]
          timeout: w288 -> [_ _ _]
          tunnel: w287 -> [w298 w299 w305]
          tunnel: [w297 w299 w304] -> w294
          tunnel: w293 -> [w296 w300 w303]
          tunnel: [w295 _ _] -> w292
          tunnel: [w296 w300 w303] -> w291
          tunnel: w286 -> [w295 _ _]
          event Timeout {
            n87 = event-data() -> ()  [unwired: 1 in, 1 out]
            n88 = call <vilib>:"Add State(s) to Queue__JKI_lib_State_Machine.vi"("State(s) in (\"\")"=w298) -> ("States Out"=w297:string)  [unwired: 14 in]
          }
          event User Event {
            # "#CSM-Example Step5.8"
            n89 = event-data() -> ()  [unwired: 1 in, 1 out]
          }
          event Panel Close? {
            n90 = event-data() -> ()  [unwired: 1 in, 1 out]
            n91 = call <vilib>:"Add State(s) to Queue__JKI_lib_State_Machine.vi"("State(s) in Front (\"\")"="Macro: Exit", "State(s) in (\"\")"=w305) -> ("States Out"=w304:string)  [unwired: 13 in]
            n92 = event-data("Discard?"=TRUE) -> ()  [unwired: 1 in, 1 out]
          }
        }
      }
      frame "CSM Documentation" {
        # "#CSM-Example Step4.2"
        # "#CSM State Syntax\n\n// Comment line, all text to the right of “//” will be ignored\n// Local Message Example\nDoSth: DoA >> Arguments\n\n// Sync Call Example\nAPI: xxxx >> Arguments -@ TargetModule\n\n// Async Call Example\nAPI: xxxx >> Arguments -> TargetModule\n\n// Async Call without Reply Example\nAPI: xxxx >> Arguments ->| TargetModule\n\n// Broadcast normal status:\nStatus >> StatusArguments  -><status>\n\n// Broadcast Interrupt status:\nInterrupt >> StatusArguments  -><interrupt>\n\n// Register Source Module's status to Handler Module\nStatus@Source Module >> Handler Module@Handler Module -><register>\n\n// Unegister Source Module's status\nStatus@Source Module >> Handler Module -><unregister>"
        # "#CSM README FIRST\n\nCSM is a LabVIEW application framework that builds upon JKI State Machine (JKISM). It follows the pattern of JKISM and extends the keywords to describe message communication between CSM modules, including concepts such as Sync-Message, Async-Message, Subscription/Unsubscription of status - essential elements for creating reusable code modules. \n\nFor more information, please visit the CSM wiki: https://github.com/NEVSTOP-LAB/JKI-State-Machine-Plus-Plus/wiki\n\nFor instructions on JKI State Machine, visit: \n    http://jki.net/state-machine/\nFor information about CSM, visit: \n    https://github.com/NEVSTOP-LAB"
      }
      frame "---------- Core ----------" {
        n93 = call <vilib>:"Add State(s) to Queue__JKI_lib_State_Machine.vi"("State(s) in (\"\")"=w313) -> ("States Out"=w312:string)  [unwired: 14 in]
      }
      frame Default {
        n94 = call "CSM Unhandled State Error.vi"("error in (no error)"=w315, "Undefined State"=w316, "CSM Name"=w317) -> ("error out"=w314:errorcluster)  [unwired: 8 in]
        n95 = call <vilib>:"Add State(s) to Queue__JKI_lib_State_Machine.vi"("State(s) in (\"\")"=w322) -> ("States Out"=w321:string)  [unwired: 14 in]
      }
      frame "VI Reference" {
        n96 = Unbundle By Name(w327) -> ("Core"=w325:T4)
        n97 = Unbundle By Name(w325) -> ("Current VI Reference"=w324:refnum<vi>)
        n98 = call "CSM - Convert Data to HexStr.vi"("Variant"=w324) -> ("HEX String (0-9,A-F)"=w323:string)  [unwired: 8 in]
      }
      frame "Error Handler" {
        # "Clear error"
        n99 = case shown="Error" w338 {
          selector: w338 -> [_ w347]
          tunnel: [w345 w349] -> w335
          tunnel: w334 -> [w345 w348]
          tunnel: [w344 w347] -> w333
          tunnel: w332 -> [w346 _]
          tunnel: w331 -> [_ _]
          tunnel: w330 -> [_ _]
          frame No Error {
            n100 = call "CSM - Convert Argument to Error.vi"("Argument"=w346) -> ("Error"=w344:errorcluster)  [unwired: 4 in]
            n101 = flat-sequence {
              frame #0 {
              }
            }
          }
          frame Error {
            n102 = call "CSM - Convert Error to Argument.vi"("Error"=w347) -> ("Argument"=w351:string)  [unwired: 4 in]
            n103 = call <vilib>:"Build State String with Arguments__JKI_lib_State_Machine.vi"("Arguments (\"\")"=w351, "State"="Error Occurred" ("Status with Arguments")) -> ("State with Arguments"=w350:string)  [unwired: 4 in]
            n104 = call "CSM - Broadcast Status Change.vi"("Status With Arguments"=w350, "State Queue"=w348) -> ("Remaining States"=w349:string)  [unwired: 13 in]
          }
        }
        n105 = disable-structure shown="Enabled" {
          disable-tunnel: w333 -> [w342 w343]
          frame Enabled {
            # "Unhandled Error -- Display it"
            n106 = call <vilib>:"General Error Handler.vi"("error in (no error)"=w342) -> ()  [unwired: 10 in, 5 out]
          }
          frame Disabled {
            n107 = call <vilib>:"Clear Errors.vi"("error in (no error)"=w343) -> ()  [unwired: 5 in, 2 out]
          }
        }
        n108 = call <vilib>:"Add State(s) to Queue__JKI_lib_State_Machine.vi"("State(s) in Front (\"\")"="// Post Error States", "State(s) in (\"\")"=w335) -> ("States Out"=w336:string)  [unwired: 13 in]
      }
      frame "Critical Error" {
        # "#CSM-Example Step5.1"
        n109 = call "CSM Critical Error.vi"("error in (no error)"=w354, "Arugments (As Reason)"=w356, "CSM Name"=w355) -> ("error out"=w353:errorcluster)  [unwired: 8 in]
        n110 = call <vilib>:"Add State(s) to Queue__JKI_lib_State_Machine.vi"("State(s) in (\"\")"=w360) -> ("States Out"=w359:string)  [unwired: 14 in]
      }
      frame "Target Timeout Error" {
        # "#CSM-Example Step5.2"
        n111 = call "CSM Target Timeout Error.vi"("error in (no error)"=w364, "Arguments (As CSM Name)"=w363) -> ("error out"=w362:errorcluster)  [unwired: 9 in]
        n112 = call <vilib>:"Add State(s) to Queue__JKI_lib_State_Machine.vi"("State(s) in (\"\")"=w368) -> ("States Out"=w367:string)  [unwired: 14 in]
      }
      frame "Target Error" {
        # "#CSM-Example Step5.3"
        n113 = call "CSM Target Error.vi"("error in (no error)"=w370, "Arguments (As CSM Name)"=w371) -> ("error out"=w369:errorcluster)  [unwired: 9 in]
        n114 = call <vilib>:"Add State(s) to Queue__JKI_lib_State_Machine.vi"("State(s) in (\"\")"=w375) -> ("States Out"=w374:string)  [unwired: 14 in]
      }
      frame "Async Response", "Response" {
        # "#CSM-Example Step5.5"
        # "#CSM-Example Step5.4"
        n115 = Unbundle(w381) -> ("‘State"=w378:string, "’Arguments"=w377:string, "’Error"=w376:errorcluster)
        n116 = case shown="Default" w378 {
          tunnel: [w388] -> w386
          tunnel: w385 -> [w389]
          tunnel: [w391] -> w384
          tunnel: w383 -> [w391]
          tunnel: [w390] -> w382
          tunnel: w376 -> [w390]
          tunnel: w380 -> [_]
          tunnel: w379 -> [_]
          tunnel: w377 -> [_]
          frame Default {
            n117 = call <vilib>:"Add State(s) to Queue__JKI_lib_State_Machine.vi"("State(s) in (\"\")"=w389) -> ("States Out"=w388:string)  [unwired: 14 in]
          }
        }
      }
      frame "Async Message Posted" {
        # "#CSM-Example Step5.6"
      }
      frame "Initialize Core Data" {
        # "originally closed?"
        # "exe?"
        # "If panel starts closed or is an EXE, then close it when we exit"
        n118 = property class="VI"() -> ("FP.State"=w398:T1)  [unwired: 2 in, 2 out]
        n119 = property class="App"() -> ("App.Kind"=w404:T2)  [unwired: 2 in, 2 out]
        n120 = control-ref of="Current VI Reference"() -> (w399:refnum<vi>)
        n121 = Equal?(x=w398, y=T1."Closed" ("Front Panel Window:State")) -> (x = y?=w396:bool)
        n122 = Equal?(x=w404, y=T2."Run Time System" ("Application:Kind")) -> (x = y?=w402:bool)
        n123 = Or(x=w396, y=w402) -> (x .or. y?=w400:bool)
        n124 = Bundle By Name(cluster=w401, "Core.Current VI Reference"=w399, "Core.Close Panel on Exit?"=w400) -> (w405:T3)
        n125 = call <vilib>:"Add State(s) to Queue__JKI_lib_State_Machine.vi"("State(s) in (\"\")"=w407) -> ("States Out"=w406:string)  [unwired: 14 in]
      }
      frame "Exit" {
        n126 = call <vilib>:"Add State(s) to Queue__JKI_lib_State_Machine.vi"("State(s) in (\"\")"=w412) -> ("States Out"=w411:string)  [unwired: 14 in]
      }
      frame "---------- Data ----------" {
        n127 = call <vilib>:"Add State(s) to Queue__JKI_lib_State_Machine.vi"("State(s) in (\"\")"=w416) -> ("States Out"=w415:string)  [unwired: 14 in]
      }
      frame "Data: Initialize" {
        w418 = T4 {"Current VI Reference"=refnum, "Close Panel on Exit?"=FALSE}  # Core
        w420 = TRUE  # Your Boolean data
        w419 = ""  # Your string data
        n128 = Bundle("Core"=w418, "Your Boolean data"=w420, "Your string data"=w419) -> (w421:T3)  [unwired: 1 in]
        n129 = call <vilib>:"Add State(s) to Queue__JKI_lib_State_Machine.vi"("State(s) in (\"\")"=w423) -> ("States Out"=w422:string)  [unwired: 14 in]
      }
      frame "Data: Cleanup" {
        n130 = Unbundle By Name(w425) -> ("Core.Current VI Reference"=w427:refnum<vi>)
        n131 = Close Reference(reference=w427) -> (error out=w426:errorcluster)  [unwired: 1 in]
        n132 = call <vilib>:"Add State(s) to Queue__JKI_lib_State_Machine.vi"("State(s) in (\"\")"=w429) -> ("States Out"=w428:string)  [unwired: 14 in]
      }
      frame "---------- Events ----------" {
        n133 = call <vilib>:"Add State(s) to Queue__JKI_lib_State_Machine.vi"("State(s) in (\"\")"=w433) -> ("States Out"=w432:string)  [unwired: 14 in]
      }
      frame "Events: Register" {
        # "#CSM-Example Step5.7"
        n134 = call "CSM - Get New State Notifier Event.vi"("Name (\"\" to Use UUID)"=w437) -> ("error out"=w435:errorcluster, "New State Notifier Event"=w436:refnum<user-event>)  [unwired: 9 in]
        n135 = register-events(error in=w435, w436) -> (reference out=w438:refnum<event-registration>, error out=w434:errorcluster)  [unwired: 1 in]
      }
      frame "Events: Unregister" {
        n136 = Unregister For Events(event registration refnum=w441) -> (error out=w442:errorcluster)  [unwired: 1 in]
      }
      frame "---------- UI ----------" {
        n137 = call <vilib>:"Add State(s) to Queue__JKI_lib_State_Machine.vi"("State(s) in (\"\")"=w448) -> ("States Out"=w447:string)  [unwired: 14 in]
      }
      frame "UI: Initialize" {
        n138 = call <vilib>:"Add State(s) to Queue__JKI_lib_State_Machine.vi"("State(s) in (\"\")"=w452) -> ("States Out"=w451:string)  [unwired: 14 in]
      }
      frame "UI: Cursor Set" {
        # "Argument"
        n139 = disable-structure shown="Default" {
          disable-tunnel: [w460 _] -> w455
          disable-tunnel: w454 -> [w459 _]
          frame condition #0 (active) {
            n140 = case shown="\"Idle\", Default" w459 {
              tunnel: [w461 w462] -> w460
              frame "Idle", Default {
                n141 = call <vilib>:"Unset Busy.vi"() -> ("error out"=w461:errorcluster)  [unwired: 11 in]
              }
              frame "Busy" {
                n142 = call <vilib>:"Set Busy.vi"() -> ("error out"=w462:errorcluster)  [unwired: 10 in, 1 out]
              }
            }
          }
          frame condition #1 {
          }
        }
        n143 = call <vilib>:"Add State(s) to Queue__JKI_lib_State_Machine.vi"("State(s) in (\"\")"=w458) -> ("States Out"=w457:string)  [unwired: 14 in]
      }
      frame "UI: Front Panel State" {
        # "Argument"
        n144 = Unbundle By Name(w466) -> ("Core.Current VI Reference"=w465:refnum<vi>)
        n145 = case shown="\"Minimize\", \"Minimized\"" w464 {
          tunnel: [w476 w489 w500 w512 w524] -> w467
          tunnel: w465 -> [w475 w487 w499 w511 w523]
          frame "Open", "Standard", Default {
            w470 = T1."Standard" ("State")
            n146 = property class="VI"(reference=w475) -> (reference out=w473:refnum<vi>, error out=w474:errorcluster, "FP.State"=w472:T1)  [unwired: 1 in]
            n147 = Not Equal?(x=w472, y=w470) -> (x != y?=w471:bool)
            n148 = case shown="True" w471 {
              tunnel: [w480 w482] -> w476
              tunnel: w474 -> [w479 w482]
              tunnel: w473 -> [w478 _]
              tunnel: w470 -> [w477 _]
              frame True {
                n149 = invoke class="VI" method="FP.Open"(reference=w478, error in=w479, "Activate"=TRUE, "State"=w477) -> (error out=w480:errorcluster)  [unwired: 1 in, 4 out]
              }
              frame False {
              }
            }
          }
          frame "Close", "Closed" {
            n150 = property class="VI"(reference=w487) -> (reference out=w486:refnum<vi>, error out=w488:errorcluster, "FP.State"=w484:T1)  [unwired: 1 in]
            n151 = Not Equal?(x=w484, y=T1."Closed" ("Front Panel Window:State")) -> (x != y?=w483:bool)
            n152 = case shown="True" w483 {
              tunnel: [w490 w493] -> w489
              tunnel: w488 -> [w490 w492]
              tunnel: w486 -> [_ w491]
              frame False {
              }
              frame True {
                n153 = invoke class="VI" method="FP.Close"(reference=w491, error in=w492) -> (error out=w493:errorcluster)  [unwired: 1 in, 2 out]
              }
            }
          }
          frame "Hidden", "Hide" {
            w494 = T1."Hidden" ("State")
            n154 = property class="VI"(reference=w499) -> (reference out=w497:refnum<vi>, error out=w498:errorcluster, "FP.State"=w496:T1)  [unwired: 1 in]
            n155 = Not Equal?(x=w496, y=w494) -> (x != y?=w495:bool)
            n156 = case shown="True" w495 {
              tunnel: [w504 w505] -> w500
              tunnel: w498 -> [w503 w505]
              tunnel: w497 -> [w502 _]
              tunnel: w494 -> [w501 _]
              frame True {
                n157 = invoke class="VI" method="FP.Open"(reference=w502, error in=w503, "State"=w501) -> (error out=w504:errorcluster)  [unwired: 2 in, 4 out]
              }
              frame False {
              }
            }
          }
          frame "Minimize", "Minimized" {
            w506 = T1."Minimized" ("State")
            n158 = property class="VI"(reference=w511) -> (reference out=w509:refnum<vi>, error out=w510:errorcluster, "FP.State"=w508:T1)  [unwired: 1 in]
            n159 = Not Equal?(x=w508, y=w506) -> (x != y?=w507:bool)
            n160 = case shown="False" w507 {
              tunnel: [w516 w517] -> w512
              tunnel: w510 -> [w515 w517]
              tunnel: w509 -> [w514 _]
              tunnel: w506 -> [w513 _]
              frame True {
                n161 = invoke class="VI" method="FP.Open"(reference=w514, error in=w515, "State"=w513) -> (error out=w516:errorcluster)  [unwired: 2 in, 4 out]
              }
              frame False {
              }
            }
          }
          frame "Maximize", "Maximized" {
            w518 = T1."Maximized" ("State")
            n162 = property class="VI"(reference=w523) -> (reference out=w521:refnum<vi>, error out=w522:errorcluster, "FP.State"=w520:T1)  [unwired: 1 in]
            n163 = Not Equal?(x=w520, y=w518) -> (x != y?=w519:bool)
            n164 = case shown="True" w519 {
              tunnel: [w528 w529] -> w524
              tunnel: w522 -> [w527 w529]
              tunnel: w521 -> [w526 _]
              tunnel: w518 -> [w525 _]
              frame True {
                n165 = invoke class="VI" method="FP.Open"(reference=w526, error in=w527, "State"=w525) -> (error out=w528:errorcluster)  [unwired: 2 in, 4 out]
              }
              frame False {
              }
            }
          }
        }
        n166 = call <vilib>:"Add State(s) to Queue__JKI_lib_State_Machine.vi"("State(s) in (\"\")"=w469) -> ("States Out"=w468:string)  [unwired: 14 in]
      }
      frame "---------- Macro ----------" {
        n167 = call <vilib>:"Add State(s) to Queue__JKI_lib_State_Machine.vi"("State(s) in (\"\")"=w533) -> ("States Out"=w532:string)  [unwired: 14 in]
      }
      frame "Macro: Initialize" {
        w535 = "Data: Initialize\nInitialize Core Data\nEvents: Register\nUI: Initialize\nUI: Front Panel State >> Open"  # Data: Initialize Initialize Core Data Events: Register UI: Initialize UI: Front Panel State >> Open
        n168 = call <vilib>:"Add State(s) to Queue__JKI_lib_State_Machine.vi"("State(s) in Front (\"\")"=w535, "State(s) in (\"\")"=w538) -> ("States Out"=w537:string)  [unwired: 13 in]
      }
      frame "Macro: Exit" {
        n169 = Unbundle By Name(w547) -> ("Core.Close Panel on Exit?"=w546:bool)
        n170 = Select(t="UI: Front Panel State >> Close", s=w546, f="") -> (s? t:f=w543:string)
        n171 = call <vilib>:"Add State(s) to Queue__JKI_lib_State_Machine.vi"("State(s) in Front (\"\")"="//Exit Sub-Modules ", "State(s) in (\"\")"=w543, "State(s) at Back (\"\")"="Data: Cleanup\nEvents: Unregister\nExit") -> ("States Out"=w541:string)  [unwired: 12 in]
        n172 = call <vilib>:"Add State(s) to Queue__JKI_lib_State_Machine.vi"("State(s) in Front (\"\")"=w541, "State(s) in (\"\")"=w549) -> ("States Out"=w548:string)  [unwired: 13 in]
      }
      frame "---------- API ----------" {
        # "#CSM-Example Step5.8"
      }
      frame "API: API1" {
      }
      frame "API: API2" {
      }
      frame "---------- Action ----------" {
        n173 = call <vilib>:"Add State(s) to Queue__JKI_lib_State_Machine.vi"("State(s) in (\"\")"=w563) -> ("States Out"=w562:string)  [unwired: 14 in]
      }
      frame "Action: action1" {
        n174 = call <vilib>:"Add State(s) to Queue__JKI_lib_State_Machine.vi"("State(s) in (\"\")"=w567) -> ("States Out"=w566:string)  [unwired: 14 in]
      }
      frame "Action: action2" {
        n175 = call <vilib>:"Add State(s) to Queue__JKI_lib_State_Machine.vi"("State(s) in (\"\")"=w571) -> ("States Out"=w570:string)  [unwired: 14 in]
      }
    }
  }
